vi "Flush Data to TXT File.vi"(8 "error in (no error)":errorcluster, 10 "queue":refnum<queue>, 11 "Logging Configuration Input":T1) -> (0 "error out":errorcluster)   [LabVIEW 2022 SP3]
doc: "Flush the data queue of any pending data and write it to the log file. Close the TDMS file reference."
uses:
  Logging Configuration.ctl
  support/TDMS-Refs.ctl
  QueuedLoggedData.ctl
  FFT-Data.ctl
  <vilib>/Waveform/WDTOps.llb/WDT Number of Waveform Samples DBL.vi
  Logging.lvlib
panel:
  out "Logging Configuration Output":T1
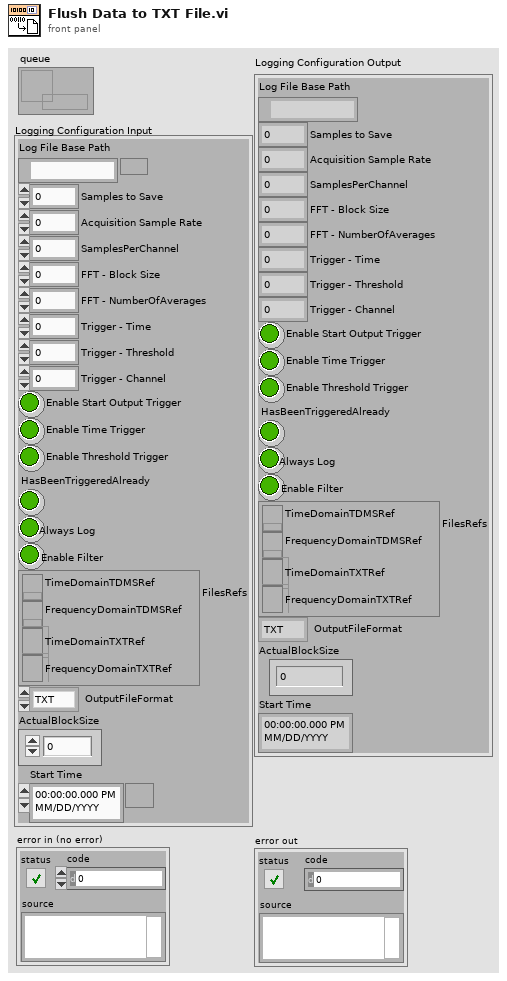
[diagram p1: front panel]
types:
  T1 = typedef "Logging.lvlib/Logging Configuration.ctl" = cluster{"Log File Base Path":path, "Samples to Save":u32, "Acquisition Sample Rate":dbl, "SamplesPerChannel":u32, "FFT - Block Size":u32, "FFT - NumberOfAverages":i32, "Trigger - Time":i32, "Trigger - Threshold":dbl, "Trigger - Channel":i32, "Enable Start Output Trigger":bool, "Enable Time Trigger":bool, "Enable Threshold Trigger":bool, "HasBeenTriggeredAlready":bool, "Always Log":bool, "Enable Filter":bool, "FilesRefs":T2, "OutputFileFormat":enum16{"TXT", "TDMS"}, "ActualBlockSize":i32, "Start Time":timestamp}
  T2 = typedef "TDMS-Refs.ctl" = cluster{"TimeDomainTDMSRef":refnum<k34>, "FrequencyDomainTDMSRef":refnum<k34>, "TimeDomainTXTRef":refnum<file>, "FrequencyDomainTXTRef ":refnum<file>}
  T3 = typedef "QueuedLoggedData.ctl" = cluster{"RawData":waveform(dbl)[], "FFT ":T4[], "Output Data":waveform(dbl)}
  T4 = typedef "FFT-Data.ctl" = cluster{"FFT-Mag":cluster{"t0":dbl, "dt":dbl, "Y":dbl[]}, "FFT-Phase":cluster{"t0":dbl, "dt":dbl, "Y":dbl[]}}
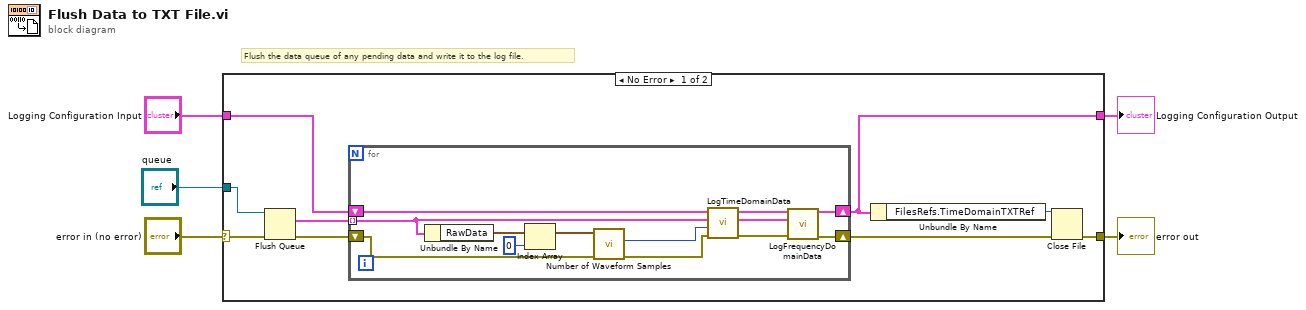
[diagram p0: block diagram]
diagram:
  # "Flush the data queue of any pending data and write it to the log file."
  n1 = case shown="No Error" "error in (no error)" {
    selector: "error in (no error)" -> [w9 w29]
    tunnel: "Logging Configuration Input" -> [w12 w28]
    tunnel: [w14 w29] -> w4
    tunnel: [w11 w28] -> w2
    tunnel: "queue" -> [w6 _]
    frame No Error {
      n2 = Flush Queue(queue=w6, error in (no error)=w9) -> (remaining elements=w7:T3[], error out=w8:errorcluster)  [unwired: 1 out]
      n3 = for {
        shift-right: [w26] -> w13
        shift-left: w8 -> [w17]
        shift-right: [w27] -> w11
        shift-left: w12 -> [w22]
        tunnel: w7 -> [w21] mode=indexing
        n4 = Unbundle By Name(w21) -> ("RawData"=w20:waveform(dbl)[])
        n5 = Index Array(array=w20, index=0) -> (element=w19:waveform(dbl))
        n6 = call-poly <vilib>:"Number of Waveform Samples.vi"("error in (no error)"=w17, "waveform in"=w19) -> ("error out"=w16:errorcluster, "number of samples"=w15:i32)  [unwired: 7 in, 1 out]
        n7 = call "LogTimeDomainData.vi"("error in (no error)"=w16, "Samples to Save In"=w15, "QueuedDataInput"=w21, "Logging Configuration"=w22) -> ("error out"=w25:errorcluster, "QueuedDataOutput"=w24:T3, "Logging Configuration Out"=w23:T1)  [unwired: 4 in, 1 out]
        n8 = call "LogFrequencyDomainData.vi"("Logging Configuration Input"=w23, "QueuedDataInput"=w24, "error in (no error)"=w25) -> ("Logging Configuration Output"=w27:T1, "error out"=w26:errorcluster)  [unwired: 11 in]
      }
      n9 = Unbundle By Name(w11) -> ("FilesRefs.TimeDomainTXTRef"=w10:refnum<file>)
      n10 = Close File(refnum=w10, error in=w13) -> (error out=w14:errorcluster)  [unwired: 1 out]
    }
    frame Error {
    }
  }
  "error out" <- w4
  "Logging Configuration Output" <- w2
